vi "Questão 2.vi"() -> ()   [LabVIEW 2019]
uses:
  <vilib>/Waveform/WDTOps.llb/WDT Get Waveform Subset DBL.vi
  <vilib>/measure/matone.llb/Extract Single Tone Information 1 Chan.vi
  <vilib>/measure/matone.llb/Extract Multiple Tone Information 1 Chan.vi
  <vilib>/measure/NI_MAPro.lvlib
panel:
  out "ONDA 8":dynamicdata(graph)
  out "ONDA 7":dynamicdata(graph)
  out "ONDA 6":dynamicdata(graph)
  out "ONDA 5":dynamicdata(graph)
  out "multiple tone information 2":T1(array[cluster]) {"detected phase (deg)" format="%_6g"; "detected amplitude" format="%_6p"; "detected frequency" format="%_6p"}
  out "ONDA TOTAL 2":waveform(dbl)(graph)
  out "waveform out":waveform(dbl)
  out "Y max":dbl format="%0.2f"
  out "Waveform Graph 2":dbl[](graph)
  out "detected frequency":dbl format="%.2p"
  out "detected amplitude":dbl format="%.2p"
  out "dt":dbl
  out "size(s)":i32
  out "Waveform Graph 4":waveform(dbl)(graph)
  in  "file path":path=path "C:/lista3.tdms"
  in  "Phase 3":dbl caption="Phase"
  in  "Amplitude 3":dbl=0.5 caption="Amplitude"
  in  "Frequency 3":dbl=40.0 caption="Frequency"
  in  "Phase 2":dbl caption="Phase"
  in  "Amplitude 2":dbl=1.0 caption="Amplitude"
  in  "Frequency 2":dbl=20.0 caption="Frequency"
  in  "Phase":dbl
  in  "Amplitude":dbl=2.0
  in  "Frequency":dbl=10.0
  out "Waveform Graph":dynamicdata(graph)
  # "Phase em graus"
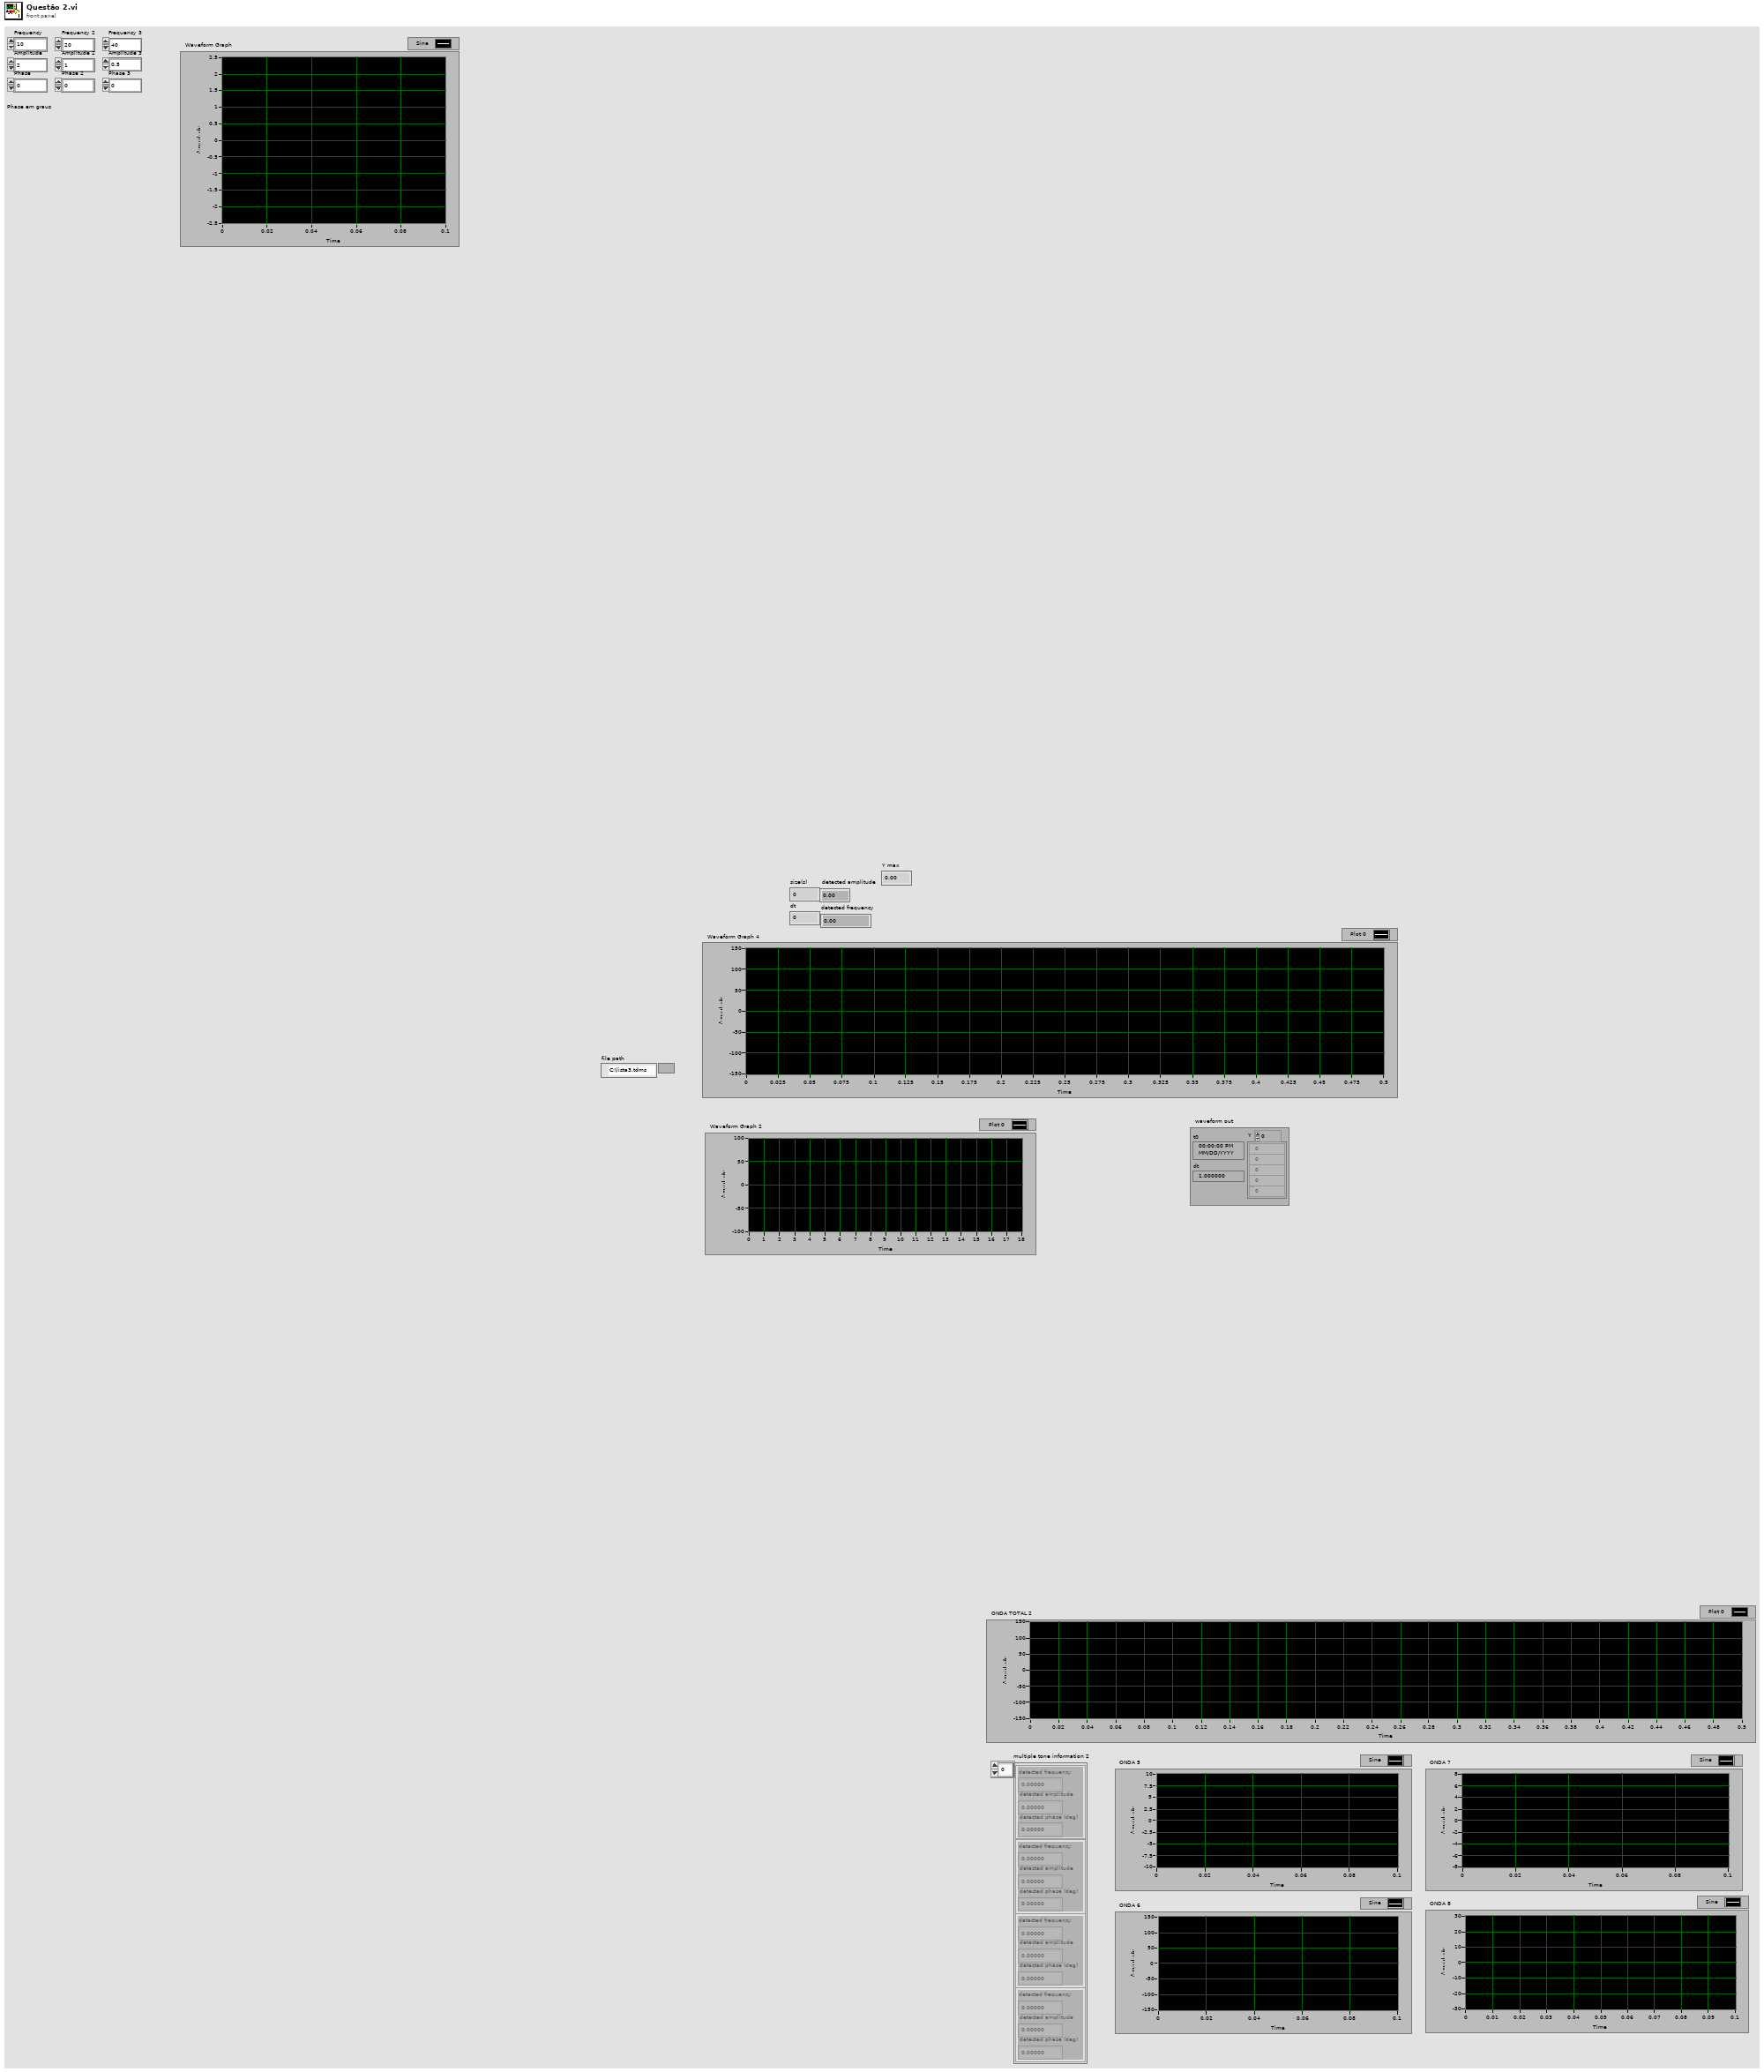
[diagram p1: front panel]
types:
  T1 = cluster{"detected frequency":dbl, "detected amplitude":dbl, "detected phase (deg)":dbl}[]
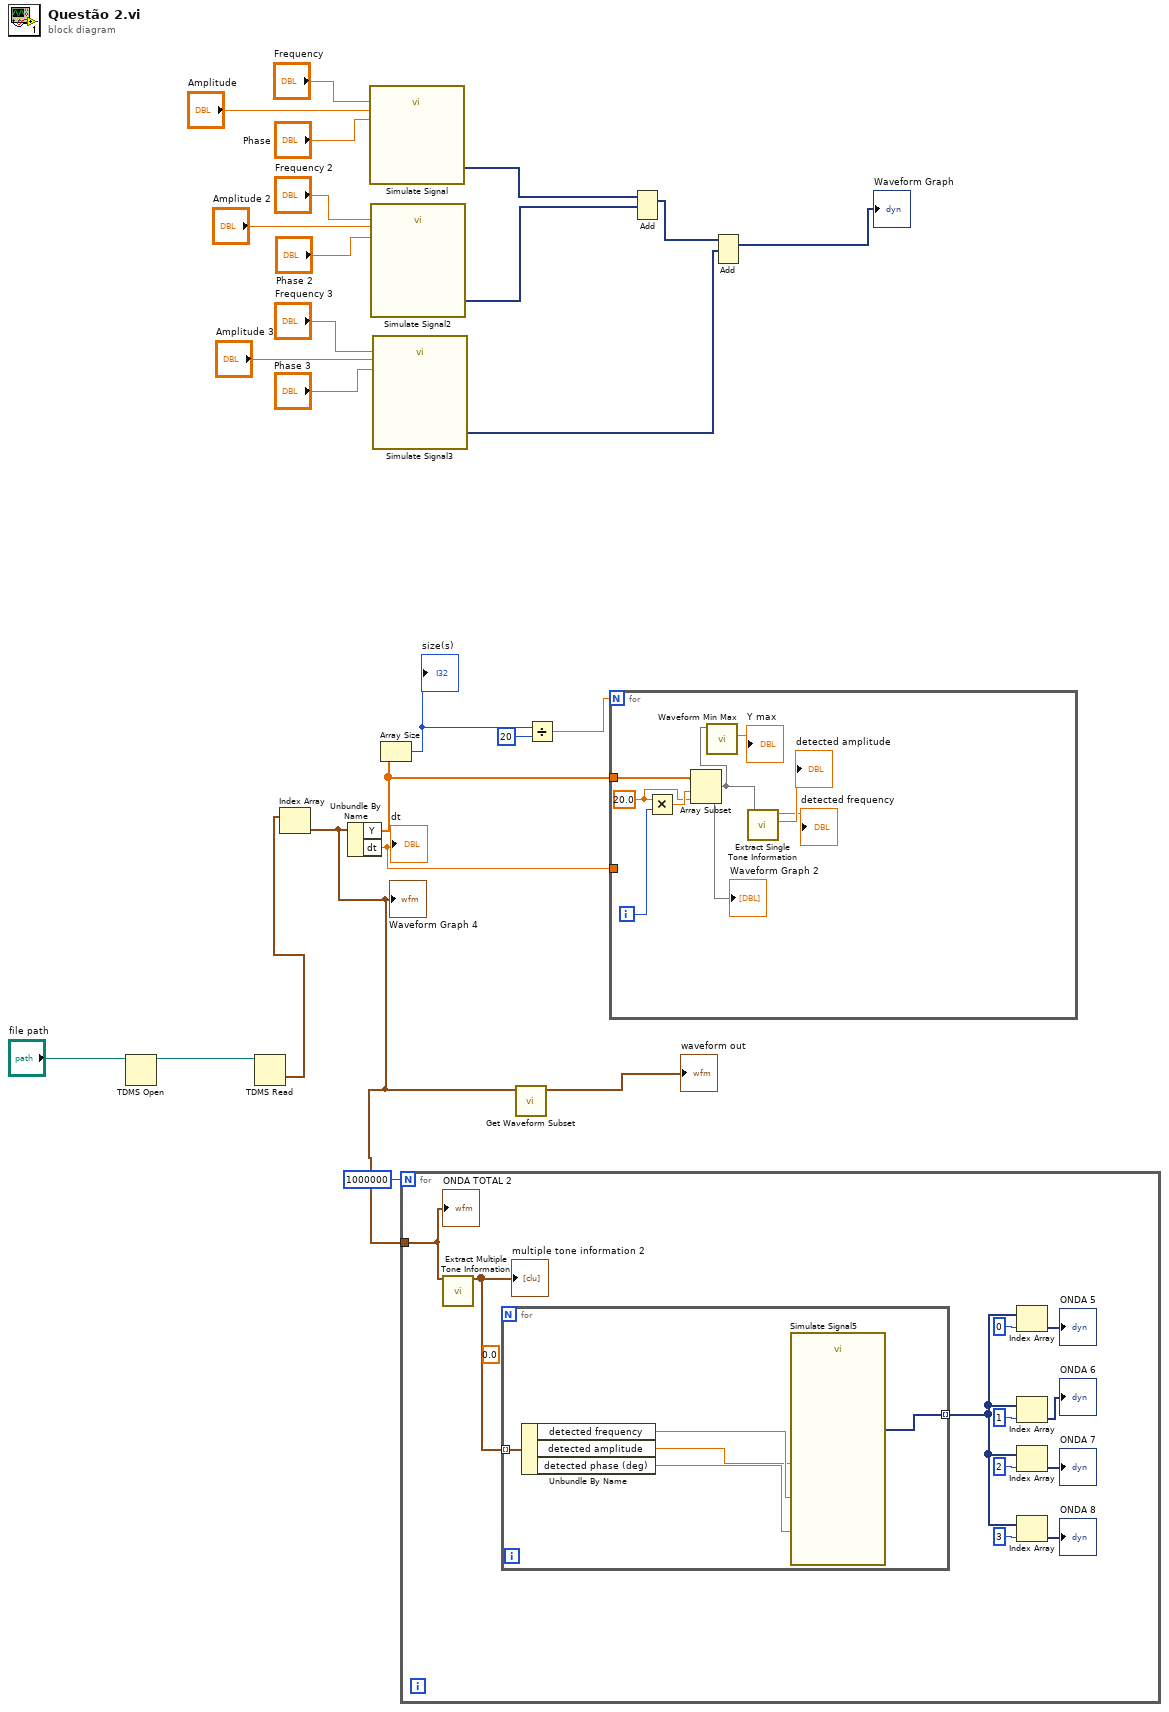
[diagram p0: block diagram]
diagram:
  n1 = TDMS Open(11:"file path") -> (3:w25:refnum<k34>)  [unwired: 6 in, 1 out]
  n2 = TDMS Read(0:w25) -> (10:w9:waveform(dbl)[])  [unwired: 7 in, 5 out]
  n3 = Index Array(array=w9) -> (element=w2:waveform(dbl))  [unwired: 1 in]
  "Waveform Graph 4" <- w2
  n4 = Unbundle By Name(w2) -> ("Y"=w5:dbl[], "dt"=w6:dbl)
  "dt" <- w6
  n5 = call "Simulate Signal"("Frequency"="Frequency", "Amplitude"="Amplitude", "Phase"="Phase") -> ("Sine"=w11:dynamicdata)  [unwired: 11 in, 1 out]
  n6 = call "Simulate Signal2"("Frequency"="Frequency 2", "Amplitude"="Amplitude 2", "Phase"="Phase 2") -> ("Sine"=w12:dynamicdata)  [unwired: 11 in, 1 out]
  n7 = call "Simulate Signal3"("Frequency"="Frequency 3", "Amplitude"="Amplitude 3", "Phase"="Phase 3") -> ("Sine"=w14:dynamicdata)  [unwired: 11 in, 1 out]
  n8 = Array Size(array=w5) -> (size(s)=w8:i32)
  "size(s)" <- w8
  n9 = for {
    N: 1000000 -> [_]
    tunnel: w2 -> [w26]
    (unwired) 0.0 ("detected amplitude")
    n10 = call-poly <vilib>:"Extract Multiple Tone Information.vi"("time signal in"=w26) -> ("multiple tone information"=w36:T1)  [unwired: 12 in, 2 out]
    "multiple tone information 2" <- w36
    n11 = for {
      tunnel: w36 -> [w41] mode=indexing
      tunnel: [w39] -> w28 mode=indexing
      n12 = Unbundle By Name(w41) -> ("detected frequency"=w40:dbl, "detected amplitude"=w37:dbl, "detected phase (deg)"=w38:dbl)
      n13 = call "Simulate Signal5"("Frequency"=w40, "Amplitude"=w37, "Phase"=w38) -> ("Sine"=w39:dynamicdata)  [unwired: 11 in, 1 out]
    }
    n14 = Index Array(array=w28, index=0) -> (element=→"ONDA 5":dynamicdata)
    n15 = Index Array(array=w28, index=1) -> (element=→"ONDA 6":dynamicdata)
    n16 = Index Array(array=w28, index=2) -> (element=→"ONDA 7":dynamicdata)
    n17 = Index Array(array=w28, index=3) -> (element=→"ONDA 8":dynamicdata)
    "ONDA TOTAL 2" <- w26
  }
  n18 = call-poly <vilib>:"Get Waveform Subset.vi"("waveform in"=w2) -> ("waveform out"=→"waveform out":waveform(dbl))  [unwired: 5 in, 3 out]
  n19 = Divide(x=w8, y=20) -> (x/y=w4:dbl)
  n20 = for {
    N: w4 -> [_]
    tunnel: w5 -> [w49]
    tunnel: w6 -> [_]
    i -> [w48]
    w46 = 20.0 ("x")
    n21 = Multiply(x=w46, y=w48) -> (x*y=w47:dbl)
    n22 = Array Subset(array=w49, index=w47, length=w46) -> (w42:dbl[])
    "Waveform Graph 2" <- w42
    n23 = call <vilib>:"Waveform Min Max.vi"("waveform in"=w42) -> ("Y max"=→"Y max":dbl)  [unwired: 5 in, 5 out]
    n24 = call-poly <vilib>:"Extract Single Tone Information.vi"("time signal in"=w42) -> ("detected amplitude"=→"detected amplitude":dbl, "detected frequency"=→"detected frequency":dbl)  [unwired: 5 in, 4 out]
  }
  n25 = Add(1:w12, 2:w11) -> (0:w13:dynamicdata)  [unwired: 1 in, 1 out]
  n26 = Add(1:w14, 2:w13) -> (0:→"Waveform Graph":dynamicdata)  [unwired: 1 in, 1 out]
